vi "Cerrar.vi"(8 "error in (no error)":errorcluster, 11 "Webcam in":refnum<class "Webcam.lvclass">) -> (0 "error out":errorcluster, 3 "Webcam out":refnum<class "Webcam.lvclass">)   [LabVIEW 2020, in "Webcam.lvclass"]
uses:
  Webcam.lvclass
  Webcam.lvclass/Webcam.ctl
  Read Session Out.vi
  Abstracta/Camara/Camara.lvclass
  <vilib>/vision/driver/NI_Vision_Acquisition_Software.lvlib
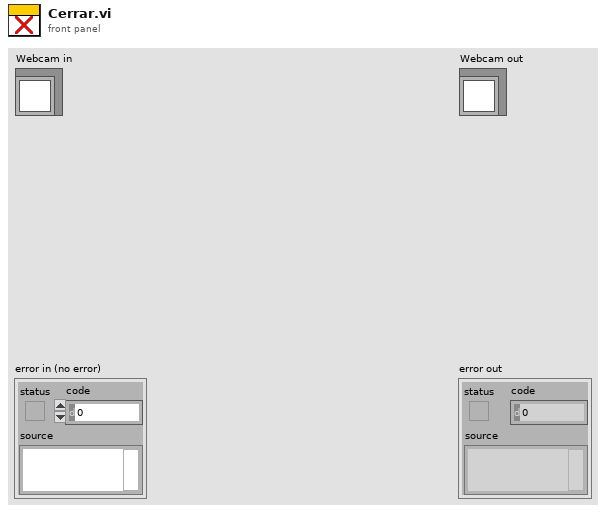
[diagram p1: front panel]
types:
  T1 = typedef "IMAQdx.ctl" = refnum<k21>
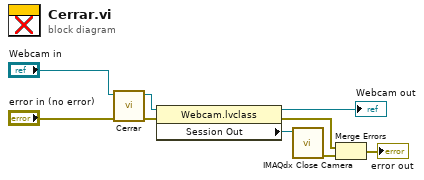
[diagram p0: block diagram]
diagram:
  n1 = call-parent "Cerrar.vi"("error in (no error)"="error in (no error)", "Camara in"="Webcam in") -> ("error out"=w9:errorcluster, "Camara out"=w5:refnum<class "Webcam.lvclass">)  [unwired: 8 in]
  n2 = property class="Webcam.lvclass"(reference=w5, error in=w9) -> (reference out=→"Webcam out":refnum<class "Webcam.lvclass">, error out=w6:errorcluster, "Session Out"=w3:T1)
  n3 = call <vilib>:"IMAQdx Close Camera.vi"("Session In"=w3) -> ("error out"=w1:errorcluster)  [unwired: 10 in]
  n4 = Merge Errors(w6, w1) -> (→"error out":errorcluster)
